vi "TestStand.Login.vi"(8 "error in":errorcluster, 11 "TS.Engine ref in":refnum<k7>) -> (0 "error out":errorcluster, 2 "success?":bool)   [LabVIEW 2019, in "Tools.lvlib"]
uses:
  Tools.lvlib
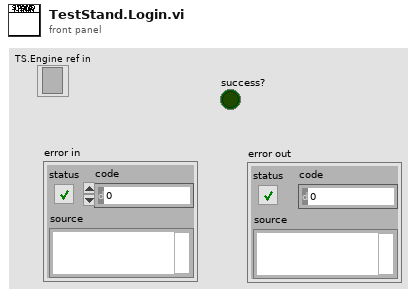
[diagram p1: front panel]
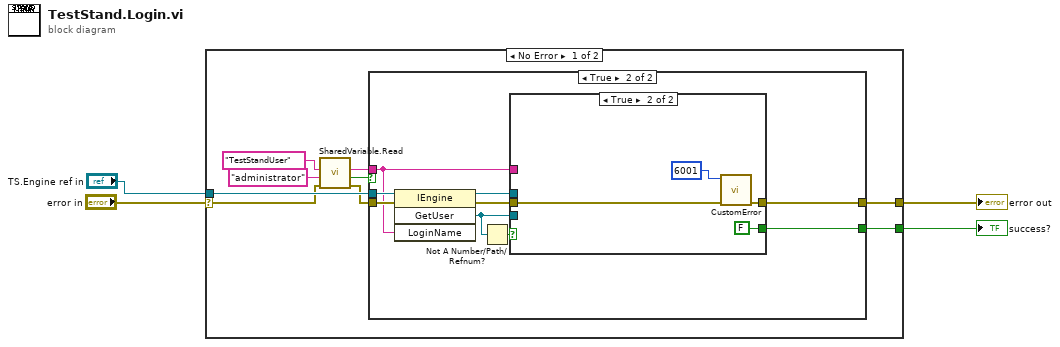
[diagram p0: block diagram]
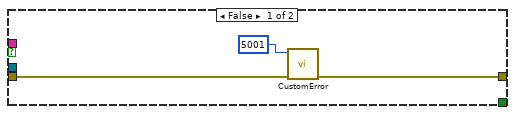
[diagram p2: hidden frame]
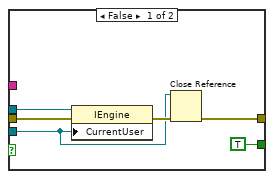
[diagram p3: hidden frame]
diagram:
  n1 = case shown="No Error" "error in" {
    selector: "error in" -> [w9 w36]
    tunnel: "TS.Engine ref in" -> [w13 _]
    tunnel: [w12 w36] -> w1
    tunnel: [w5 _] -> w4
    frame No Error {
      n2 = call "SharedVariable.Read.vi"("error in"=w9, "default value"="administrator", "variable"="TestStandUser") -> ("error out"=w8:errorcluster, "found"=w6:bool, "value"=w7:string)  [unwired: 6 in]
      n3 = case shown="True" w6 {
        tunnel: w13 -> [_ w25]
        tunnel: [w14 w19] -> w12
        tunnel: w8 -> [w15 w22]
        tunnel: w7 -> [_ w21]
        tunnel: [_ w20] -> w5
        frame False {
          n4 = call "CustomError.vi"("Error In"=w15, "Error code"=5001 ("error code (0)")) -> ("Error Out"=w14:errorcluster)  [unwired: 9 in]
        }
        frame True {
          n5 = invoke class="IEngine" method="GetUser"(reference=w25, error in=w22, "LoginName"=w21) -> (reference out=w23:refnum<k7>, error out=w24:errorcluster, "GetUser"=w18:refnum<k7>)  [unwired: 1 in, 1 out]
          n6 = Not A Number/Path/Refnum?(number/path/refnum=w18) -> (NaN/Path/Refnum?=w17:bool)
          n7 = case shown="True" w17 {
            tunnel: w24 -> [w31 w35]
            tunnel: [w27 w34] -> w19
            tunnel: w23 -> [w30 _]
            tunnel: w18 -> [w28 _]
            tunnel: w21 -> [_ _]
            tunnel: [TRUE FALSE] -> w20
            frame False {
              n8 = property class="IEngine"(reference=w30, error in=w31, "CurrentUser"=w28) -> (error out=w29:errorcluster)  [unwired: 1 out]
              n9 = Close Reference(reference=w28, error in (no error)=w29) -> (error out=w27:errorcluster)
            }
            frame True {
              n10 = call "CustomError.vi"("Error In"=w35, "Error code"=6001 ("error code (0)")) -> ("Error Out"=w34:errorcluster)  [unwired: 9 in]
            }
          }
        }
      }
    }
    frame Error {
    }
  }
  "error out" <- w1
  "success?" <- w4
